vi "Workspace.UI.Update.vi"(7 "Diagnostic Protocol":T1, 8 "error in (no error)":errorcluster, 9 "Data.PendingChange?":bool, 10 "Values":dbl[](array[numeric]), 11 "UI.Refs":T2) -> (0 "error out":errorcluster)   [LabVIEW 2019, in "Diagnostics Addon Shared.lvlib"]
uses:
  Diagnostics Addon Shared.lvlib
  Types/UI.Refs.ctl
  Types/Command.ctl
  Types/Protocol.ctl
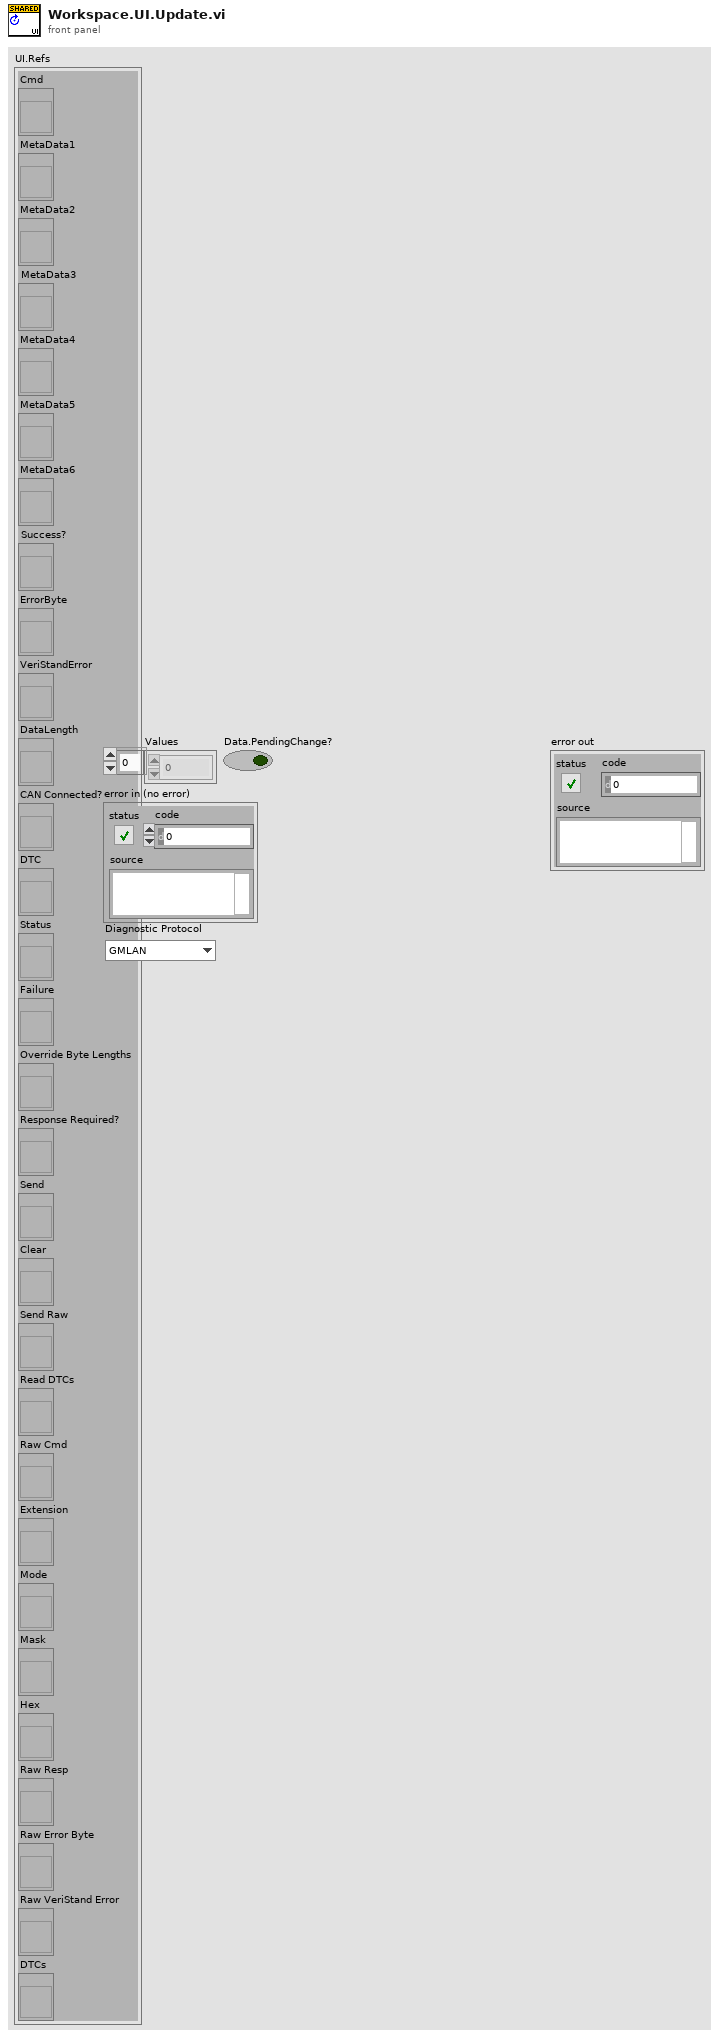
[diagram p1: front panel]
types:
  T1 = typedef "Diagnostics Addon Shared.lvlib/Protocol.ctl" = enum16{"GMLAN", "KWP-2000", "UDS", "User-Defined"}
  T2 = typedef "Diagnostics Addon Shared.lvlib/UI.Refs.ctl" = cluster{"Cmd":refnum<vi>, "MetaData1":refnum<vi>, "MetaData2":refnum<vi>, "MetaData3":refnum<vi>, "MetaData4":refnum<vi>, "MetaData5":refnum<vi>, "MetaData6":refnum<vi>, "Success?":refnum<vi>, "ErrorByte":refnum<vi>, "VeriStandError":refnum<vi>, "DataLength":refnum<vi>, "CAN Connected?":refnum<vi>, "DTC":refnum<vi>, "Status":refnum<vi>, "Failure":refnum<vi>, "Override Byte Lengths":refnum<vi>, "Response Required?":refnum<vi>, "Send":refnum<vi>, "Clear":refnum<vi>, "Send Raw":refnum<vi>, "Read DTCs":refnum<vi>, "Raw Cmd":refnum<vi>, "Extension":refnum<vi>, "Mode":refnum<vi>, "Mask":refnum<vi>, "Hex":refnum<vi>, "Raw Resp":refnum<vi>, "Raw Error Byte":refnum<vi>, "Raw VeriStand Error":refnum<vi>, "DTCs":refnum<vi>}
  T3 = typedef "Diagnostics Addon Shared.lvlib/Command.ctl" = enum8{"None", "EnableDiagnosticSession", "DisableDiagnosticSession", "ReadDataIdentifiers", "ReadDataIdentifier", "WriteDataIndentifier", "ReadPIDsOnDemand", "ReadPIDOnDemand", "WriteCPID", "WriteMemory", "ReadMemory", "ReadDTCs", "ClearDTCs", "ControlDTC", "ForceTesterPresent", "DisableNormalCommunication", "ReturnToNormalMode", "InputOutputControl", "StartRoutine", "RequestRoutineStatus", "StopRoutine", "ECUReset", "UnlockECU", "ClearSuccessBit", "ConfigureandStartPIDs", "StopPIDs", "StartDTCs", "EnableChangeDTCCount", "DisableChangeDTCCount", "ReadFailureRecordParameters", "PassThru Channel Based", "EnableRepeatingTesterPresent", "DisableRepeatingTesterPresent", "CloseCANCommunication", "RestartCANCommunication"}
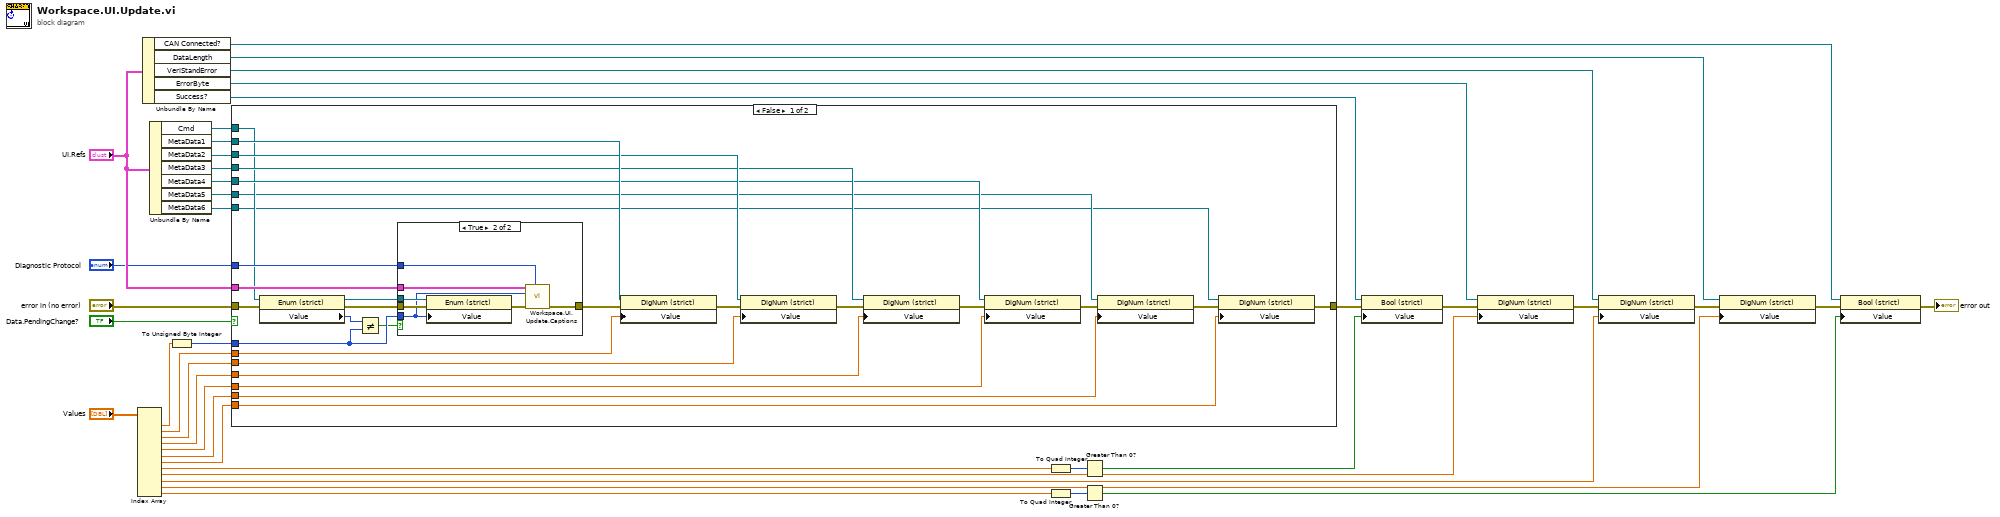
[diagram p0: block diagram]
diagram:
  n1 = Index Array(array="Values") -> (element #1=w31:dbl, element #2=w30:dbl, element #3=w29:dbl, element #4=w28:dbl, element #5=w27:dbl, element #6=w2:dbl, element #7=w1:dbl, element #8=w3:dbl, element #9=w4:dbl, element #10=w5:dbl, element #11=w6:dbl, element #12=w7:dbl)  [unwired: 12 in]
  n2 = Unbundle By Name("UI.Refs") -> ("CAN Connected?"=w12:refnum<vi>, "DataLength"=w16:refnum<vi>, "VeriStandError"=w17:refnum<vi>, "ErrorByte"=w18:refnum<vi>, "Success?"=w19:refnum<vi>)
  n3 = Unbundle By Name("UI.Refs") -> ("Cmd"=w23:refnum<vi>, "MetaData1"=w38:refnum<vi>, "MetaData2"=w37:refnum<vi>, "MetaData3"=w36:refnum<vi>, "MetaData4"=w35:refnum<vi>, "MetaData5"=w9:refnum<vi>, "MetaData6"=w8:refnum<vi>)
  n4 = To Unsigned Byte Integer(number=w31) -> (unsigned 8bit integer=w22:u8)
  n5 = case shown="False" "Data.PendingChange?" {
    tunnel: w38 -> [w68 _]
    tunnel: w37 -> [w67 _]
    tunnel: w36 -> [w66 _]
    tunnel: w35 -> [w62 _]
    tunnel: [w45 w77] -> w34
    tunnel: w30 -> [w60 _]
    tunnel: w29 -> [w59 _]
    tunnel: w28 -> [w58 _]
    tunnel: w27 -> [w57 _]
    tunnel: "error in (no error)" -> [w56 w77]
    tunnel: w23 -> [w49 _]
    tunnel: w22 -> [w53 _]
    tunnel: "UI.Refs" -> [w51 _]
    tunnel: "Diagnostic Protocol" -> [w50 _]
    tunnel: w9 -> [w44 _]
    tunnel: w8 -> [w43 _]
    tunnel: w2 -> [w42 _]
    tunnel: w1 -> [w41 _]
    frame False {
      n6 = property class="Enum (strict)"(reference=w49, error in=w56) -> (reference out=w48:refnum<vi>, error out=w55:errorcluster, "Value"=w54:T3)
      n7 = Not Equal?(x=w54, y=w53) -> (x != y?=w52:bool)
      n8 = case shown="True" w52 {
        tunnel: [w69 w73] -> w65
        tunnel: w55 -> [w69 w76]
        tunnel: w48 -> [_ w75]
        tunnel: w53 -> [_ w72]
        tunnel: w51 -> [_ w71]
        tunnel: w50 -> [_ w70]
        frame False {
        }
        frame True {
          n9 = property class="Enum (strict)"(reference=w75, error in=w76, "Value"=w72) -> (error out=w74:errorcluster)  [unwired: 1 out]
          n10 = call "Workspace.UI.Update.Captions.vi"("Diagnostic Protocol"=w70, "error in (no error)"=w74, "Cmd"=w72, "UI.Refs"=w71) -> ("error out"=w73:errorcluster)  [unwired: 7 in]
        }
      }
      n11 = property class="DigNum (strict)"(reference=w68, error in=w65, "Value"=w60) -> (error out=w64:errorcluster)  [unwired: 1 out]
      n12 = property class="DigNum (strict)"(reference=w67, error in=w64, "Value"=w59) -> (error out=w63:errorcluster)  [unwired: 1 out]
      n13 = property class="DigNum (strict)"(reference=w66, error in=w63, "Value"=w58) -> (error out=w61:errorcluster)  [unwired: 1 out]
      n14 = property class="DigNum (strict)"(reference=w62, error in=w61, "Value"=w57) -> (error out=w46:errorcluster)  [unwired: 1 out]
      n15 = property class="DigNum (strict)"(reference=w44, error in=w46, "Value"=w42) -> (error out=w47:errorcluster)  [unwired: 1 out]
      n16 = property class="DigNum (strict)"(reference=w43, error in=w47, "Value"=w41) -> (error out=w45:errorcluster)  [unwired: 1 out]
    }
    frame True {
    }
  }
  n17 = To Quad Integer(1:w3) -> (0:w25:i64)
  n18 = To Quad Integer(1:w7) -> (0:w11:i64)
  n19 = Greater Than 0?(x=w25) -> (x > 0?=w26:bool)
  n20 = Greater Than 0?(x=w11) -> (x > 0?=w10:bool)
  n21 = property class="Bool (strict)"(reference=w19, error in=w34, "Value"=w26) -> (error out=w33:errorcluster)  [unwired: 1 out]
  n22 = property class="DigNum (strict)"(reference=w18, error in=w33, "Value"=w4) -> (error out=w39:errorcluster)  [unwired: 1 out]
  n23 = property class="DigNum (strict)"(reference=w17, error in=w39, "Value"=w5) -> (error out=w40:errorcluster)  [unwired: 1 out]
  n24 = property class="DigNum (strict)"(reference=w16, error in=w40, "Value"=w6) -> (error out=w14:errorcluster)  [unwired: 1 out]
  n25 = property class="Bool (strict)"(reference=w12, error in=w14, "Value"=w10) -> (error out=→"error out":errorcluster)  [unwired: 1 out]
